vi "Extra 1.vi"(8 "error in (no error)":errorcluster, 11 "Node Ptr":T1 format="%.0x") -> (0 "error out":errorcluster)   [LabVIEW 2017, in "Data Sharing Custom Device System Explorer.lvlib"]
uses:
  Data Sharing Custom Device System Explorer.lvlib
  <vilib>/NI Veristand/Custom Device API/Custom Device Item Ref.ctl
  <vilib>/NI VeriStand/Custom Device API/Custom Device API.lvlib
panel:
  in  "SHDocVw.IWebBrowser":refnum<k7>(container)
  in  "Specific Header":cluster{"Section Name":string}={"Section Name"="Specific Page Settings"}
  in  "General Header":cluster{"Section Name":string}={"Section Name"="General Page Settings"}
  in  "Description":string
  in  "Name":string
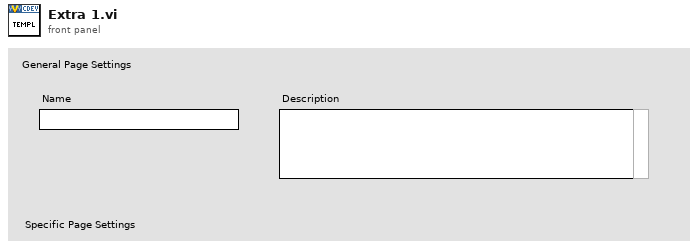
[diagram p1: front panel]
types:
  T1 = typedef "Custom Device API.lvlib/Custom Device Item Ref.ctl" = u64
  T2 = typedef "Custom Device API.lvlib/Custom Device Item Info.ctl" = cluster{"Name":string, "Is Channel":bool, "GUID":string, "Is Waveform":bool}
  T3 = typedef "Custom Device API.lvlib/Custom Device Commands.ctl" = enum16{"Default", "Item renamed", "Shutdown", "Dynamic button pressed"}
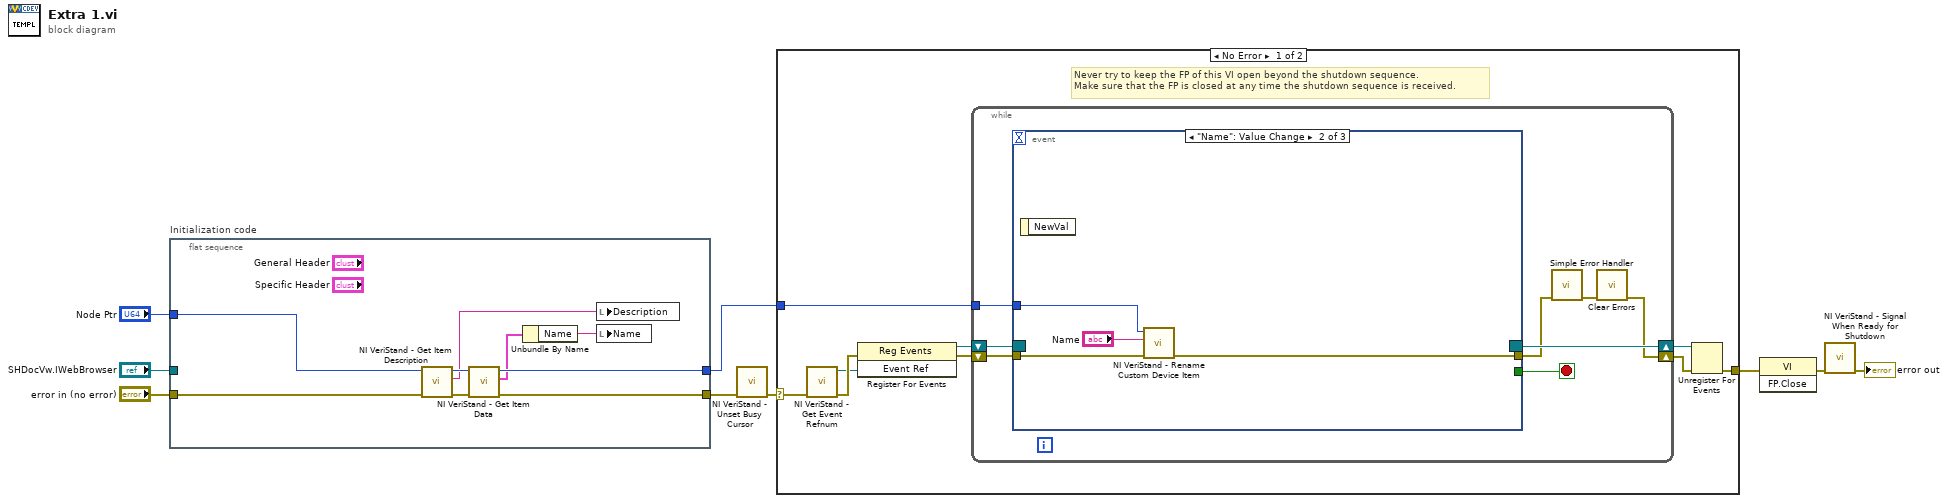
[diagram p0: block diagram]
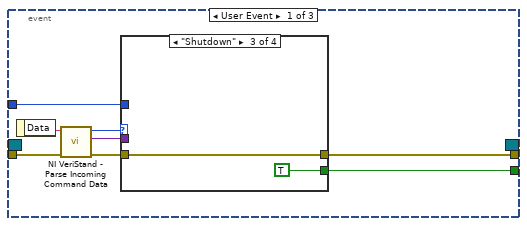
[diagram p2: hidden frame]
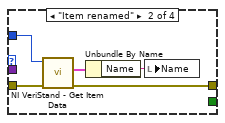
[diagram p4: hidden frame]
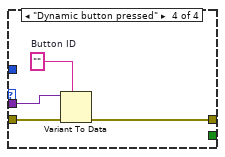
[diagram p5: hidden frame]
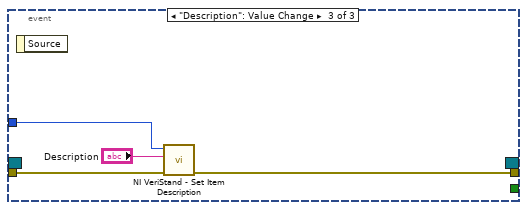
[diagram p6: hidden frame]
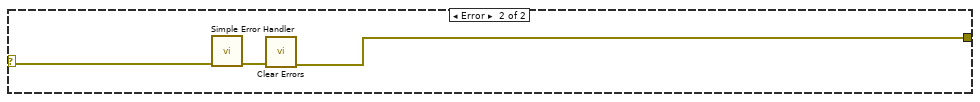
[diagram p7: hidden frame]
diagram:
  n1 = flat-sequence "Initialization code" {
    tunnel: "error in (no error)" -> [w10]
    tunnel: "Node Ptr" -> [w13]
    tunnel: [w14] -> w5
    tunnel: [w18] -> w2
    tunnel: "SHDocVw.IWebBrowser" -> [_]
    frame #0 {
      n2 = call <vilib>:"NI VeriStand - Get Item Description.vi"("error in (no error)"=w10, "Item Ref in"=w13) -> ("error out"=w16:errorcluster, "Description"=w11:string, "Item Ref out"=w17:T1)  [unwired: 7 out]
      n3 = call <vilib>:"NI VeriStand - Get Item Data.vi"("error in (no error)"=w16, "Item Ref in"=w17) -> ("error out"=w14:errorcluster, "Item Info"=w15:T2, "Item Ref out"=w18:T1)  [unwired: 7 out]
      n4 = Unbundle By Name(w15) -> ("Name"=w12:string)
      n5 = local write "Description"(w11) -> ()
      n6 = local write "Name"(w12) -> ()
    }
  }
  n7 = call <vilib>:"NI VeriStand - Unset Busy Cursor.vi"("error in (no error)"=w5) -> ("error out"=w4:errorcluster)  [unwired: 10 out]
  n8 = case shown="No Error" w4 {
    selector: w4 -> [w19 w66]
    tunnel: [w24 w64] -> w9
    tunnel: w2 -> [w20 _]
    frame No Error {
      # "Never try to keep the FP of this VI open beyond the shutdown sequence.\nMake sure that the FP is closed at any time the shutdown sequence is received."
      n9 = call <vilib>:"NI VeriStand - Get Event Refnum.vi"("error in (no error)"=w19) -> ("error out"=w27:errorcluster, "Event Ref"=w23:refnum<user-event>)  [unwired: 9 out]
      n10 = register-events(error in=w27, w23) -> (reference out=w21:refnum<event-registration>, error out=w22:errorcluster)  [unwired: 1 in]
      n11 = while {
        tunnel: w20 -> [w31]
        shift-right: [w28] -> w25
        shift-left: w22 -> [w34]
        shift-right: [w35] -> w26
        shift-left: w21 -> [w33]
        stop <- w32 stop-if-true
        n12 = event shown="[1] \"Name\": Value Change" {
          selector: w33 -> [_ _ _]
          dyn-events: [_ _ _] -> w35
          timeout: _ -> [_ _ _]
          tunnel: w34 -> [w43 w59 w62]
          tunnel: [w39 _ _] -> w32
          tunnel: [w38 w58 w61] -> w30
          tunnel: w31 -> [w37 w57 w63]
          event User Event {
            n13 = event-data() -> ("Data"=w42:string)  [unwired: 1 out]
            n14 = call <vilib>:"NI VeriStand - Parse Incoming Command Data.vi"("error in (no error)"=w43, "Incoming data"=w42) -> ("error out"=w41:errorcluster, "Outgoing data"=w36:variant, "Action"=w40:T3)  [unwired: 7 out]
            n15 = case shown="\"Shutdown\"" w40 {
              tunnel: w41 -> [w44 w49 w50 w55]
              tunnel: [_ _ TRUE _] -> w39
              tunnel: [w44 w46 w50 w52] -> w38
              tunnel: w37 -> [_ w48 _ _]
              tunnel: w36 -> [_ _ _ w54]
              frame "Default", Default {
              }
              frame "Item renamed" {
                n16 = call <vilib>:"NI VeriStand - Get Item Data.vi"("error in (no error)"=w49, "Item Ref in"=w48) -> ("error out"=w46:errorcluster, "Item Info"=w47:T2)  [unwired: 8 out]
                n17 = Unbundle By Name(w47) -> ("Name"=w45:string)
                n18 = local write "Name"(w45) -> ()
              }
              frame "Shutdown" {
              }
              frame "Dynamic button pressed" {
                w53 = ""  # Button ID
                n19 = Variant To Data(error in=w55, type=w53, Variant=w54) -> (error out=w52:errorcluster)  [unwired: 1 out]
              }
            }
          }
          event "Name": Value Change {
            n20 = event-data() -> ()  [unwired: 2 out]
            n21 = call <vilib>:"NI VeriStand - Rename Custom Device Item.vi"("error in (no error)"=w59, "New Name"="Name", "Item Ref in"=w57) -> ("error out"=w58:errorcluster)  [unwired: 1 in, 7 out]
          }
          event "Description": Value Change {
            n22 = event-data() -> ()  [unwired: 2 out]
            n23 = call <vilib>:"NI VeriStand - Set Item Description.vi"("error in (no error)"=w62, "Description"="Description", "Item Ref in"=w63) -> ("error out"=w61:errorcluster)  [unwired: 8 out]
          }
        }
        n24 = call <vilib>:"Simple Error Handler.vi"("error in (no error)"=w30) -> ("error out"=w29:errorcluster)  [unwired: 1 in, 7 out]
        n25 = call <vilib>:"Clear Errors.vi"("error in (no error)"=w29) -> ("error out"=w28:errorcluster)  [unwired: 1 in, 5 out]
      }
      n26 = Unregister For Events(event registration refnum=w26, error in=w25) -> (error out=w24:errorcluster)
    }
    frame Error {
      n27 = call <vilib>:"Simple Error Handler.vi"("error in (no error)"=w66) -> ("error out"=w65:errorcluster)  [unwired: 1 in, 7 out]
      n28 = call <vilib>:"Clear Errors.vi"("error in (no error)"=w65) -> ("error out"=w64:errorcluster)  [unwired: 1 in, 5 out]
    }
  }
  n29 = invoke class="VI" method="FP.Close"(error in=w9) -> (error out=w8:errorcluster)  [unwired: 2 in, 2 out]
  n30 = call <vilib>:"NI VeriStand - Signal When Ready for Shutdown.vi"("error in (no error)"=w8) -> ("error out"=→"error out":errorcluster)  [unwired: 10 out]
